vi "Module_Close_SMU's.vi"(8 "Error In":errorcluster, 11 "Instrument_Visas":T1={"DUT and Bridge Power"="4145_0", "Throw_Meas"="4139_1"}) -> (0 "Error Out":errorcluster)   [LabVIEW 2013]
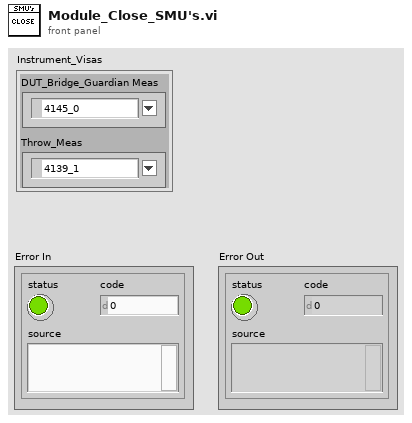
[diagram p1: front panel]
types:
  T1 = cluster{"DUT and Bridge Power":refnum<k15>, "Throw_Meas":refnum<k15>}
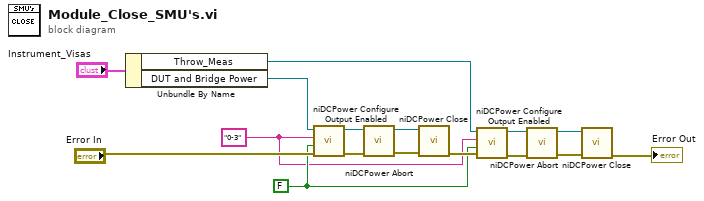
[diagram p0: block diagram]
diagram:
  w4 = "0-3" ("channel name")
  w5 = FALSE ("output enabled")
  n1 = Unbundle By Name("Instrument_Visas") -> ("Throw_Meas"=w9:refnum<k15>, "DUT and Bridge Power"=w10:refnum<k15>)
  n2 = call <instrlib>:"niDCPower Configure Output Enabled.vi"("error in (no error)"="Error In", "output enabled"=w5, "channel name"=w4, "instrument handle"=w10) -> ("error out"=w13:errorcluster, "instrument handle out"=w8:refnum<k15>)  [unwired: 6 in]
  n3 = call <instrlib>:"niDCPower Abort.vi"("error in (no error)"=w13, "instrument handle"=w8) -> ("error out"=w12:errorcluster, "instrument handle out"=w7:refnum<k15>)  [unwired: 8 in]
  n4 = call <instrlib>:"niDCPower Close.vi"("error in (no error)"=w12, "instrument handle"=w7) -> ("error out"=w11:errorcluster)  [unwired: 9 in]
  n5 = call <instrlib>:"niDCPower Configure Output Enabled.vi"("error in (no error)"=w11, "output enabled"=w5, "channel name"=w4, "instrument handle"=w9) -> ("error out"=w16:errorcluster, "instrument handle out"=w3:refnum<k15>)  [unwired: 6 in]
  n6 = call <instrlib>:"niDCPower Abort.vi"("error in (no error)"=w16, "instrument handle"=w3) -> ("error out"=w15:errorcluster, "instrument handle out"=w2:refnum<k15>)  [unwired: 8 in]
  n7 = call <instrlib>:"niDCPower Close.vi"("error in (no error)"=w15, "instrument handle"=w2) -> ("error out"=→"Error Out":errorcluster)  [unwired: 9 in]
